vi "Phase_calculator_one_mask.vi"(9 "User-defined phase":dbl=4.0 format="%#_13g", 10 "User-defined Amplitude":dbl=0.3, 11 "Pixel":dbl=400.0) -> (0 "Voltage B Output":dbl=3921.0, 3 "Voltage A Output":dbl=1204.0)   [LabVIEW 2016]
uses:
  <vilib>/Utility/file.llb/Read Delimited Spreadsheet (DBL).vi
panel:
  out "Phase B Output 2":dbl=2.961 format="%#_8g"
  out "Voltage B Output 2":dbl=3921.0
  out "Amplitude Output 2":dbl=0.27793470017986477
  out "Phase Output 2":dbl=3.9764999999999997
  out "Voltage A Output 2":dbl=1204.0
  out "Phase A Output 2":dbl=4.992 format="%#_8g"
  in  "User-defined  Phi B":dbl=0.3
  out "arccos(A) 2":dbl=0.9911565864311924
  in  "User-defined Amplitude 2":dbl=0.3
  in  "Mask B phase output":cluster{"all rows":dbl[], "all rows":dbl[]}
  in  "Mask A phase output":cluster{"all rows":dbl[], "all rows":dbl[]}
  out "Amplitude Output":dbl=0.27793470017986477
  out "Phase Output":dbl=3.9764999999999997
  out "Phase A Output":dbl=4.992 format="%#_8g"
  out "Phase B Output":dbl=2.961 format="%#_8g"
  out "arccos(A)":dbl=0.9911565864311924
  in  "Mask B data string":string="G:\\My Drive\\ansom\\Data\\THz 1\\pulse shaping\\SLM calibration 5 August 2021\\Mask_B_phase_voltage\\Mask_B_phase_pixel_"
  in  "Mask A data string":string="G:\\My Drive\\ansom\\Data\\THz 1\\pulse shaping\\SLM calibration 5 August 2021\\Mask_A_phase_voltage\\Mask_A_phase_pixel_"
  out "Mask B Phase":cluster{"Ramp Pattern":dbl[], "phase out":dbl[]}(graph)
  out "Mask A Phase":cluster{"Ramp Pattern":dbl[], "phase out":dbl[]}(graph)
  in  "OK":bool
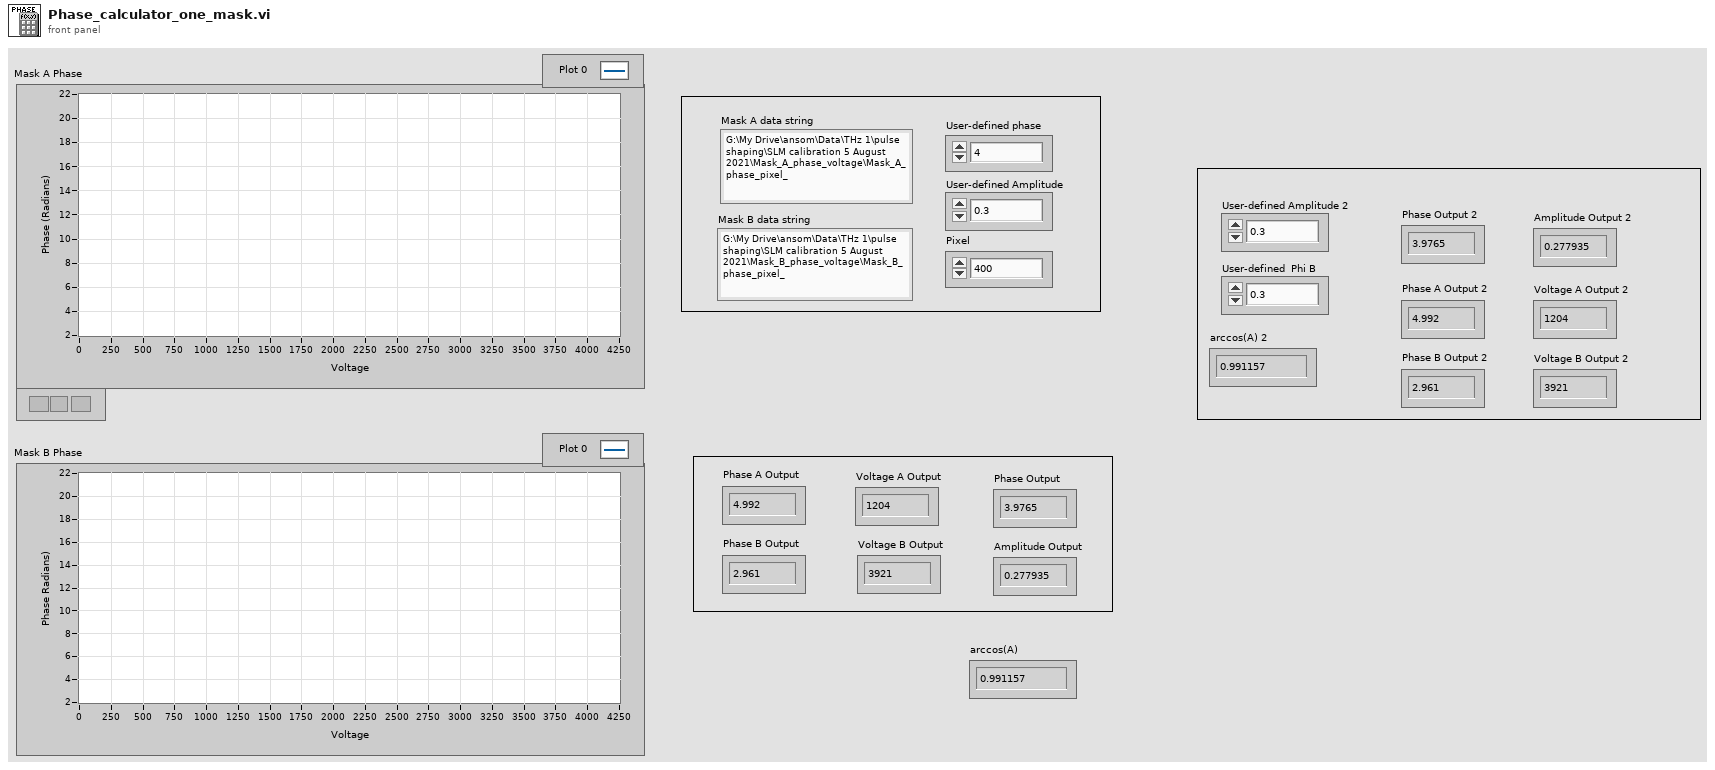
[diagram p1: front panel]
types:
  T1 = enum32{"Invalid", "Standard", "Closed", "Hidden", "Minimized", "Maximized"}
  T2 = enum32{"invalid app kind", "Development System", "Run Time System", "Student Edition", "Embedded LabVIEW", "Evaluation", "Custom"}
  T3 = cluster{"Core":cluster{"Current VI Reference":refnum<vi>, "Close Panel on Exit?":bool}, "Mask A phase output":cluster{"all rows":dbl[], "all rows":dbl[]}, "Mask B phase output":cluster{"all rows":dbl[], "all rows":dbl[]}}
  T4 = cluster{"Current VI Reference":refnum<vi>, "Close Panel on Exit?":bool}
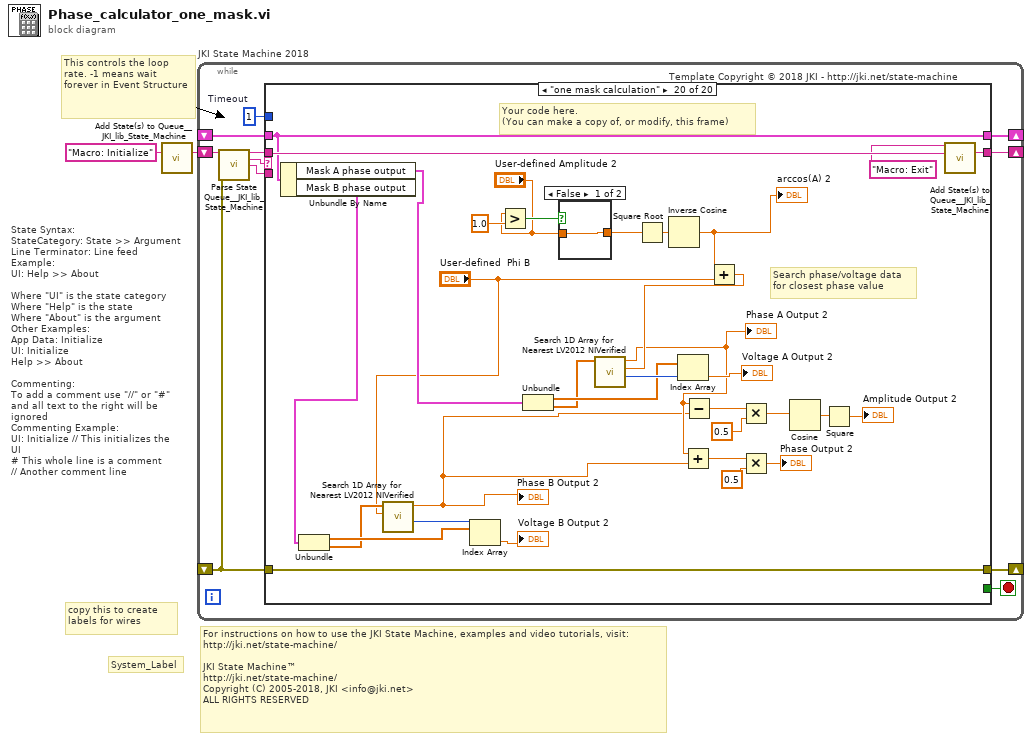
[diagram p0: block diagram]
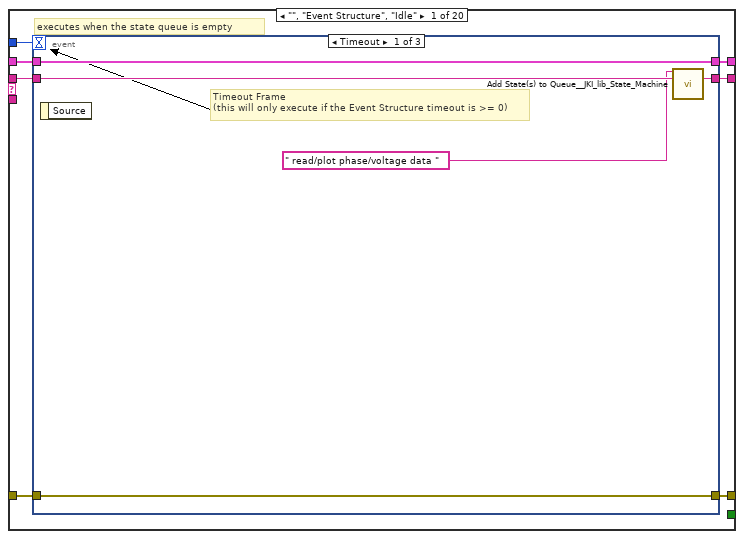
[diagram p2: hidden frame]
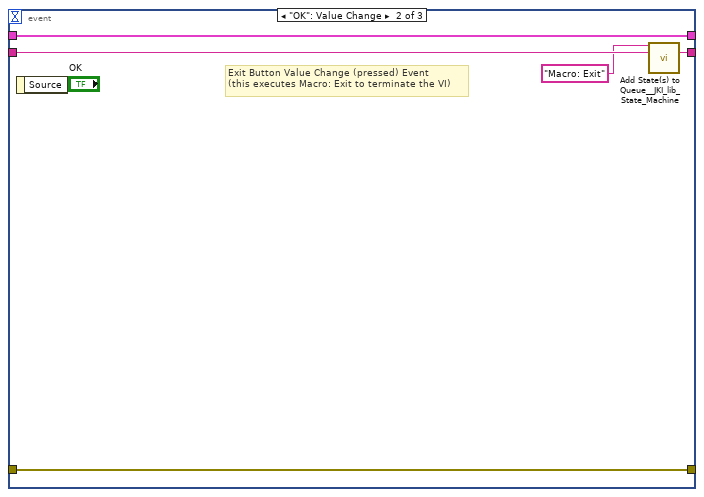
[diagram p3: hidden frame]
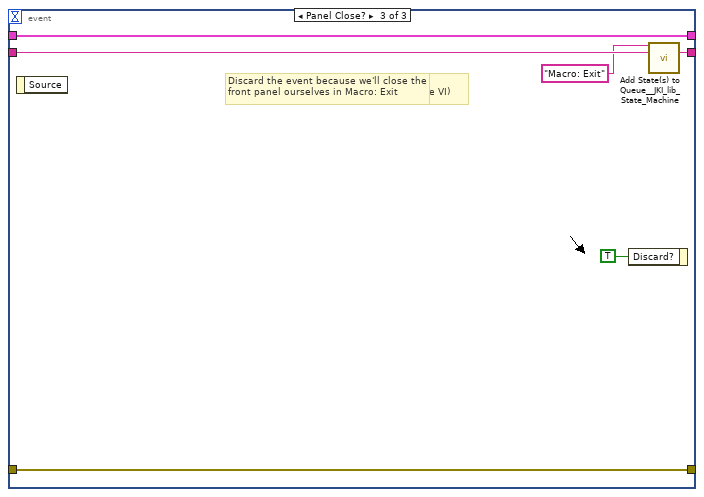
[diagram p4: hidden frame]
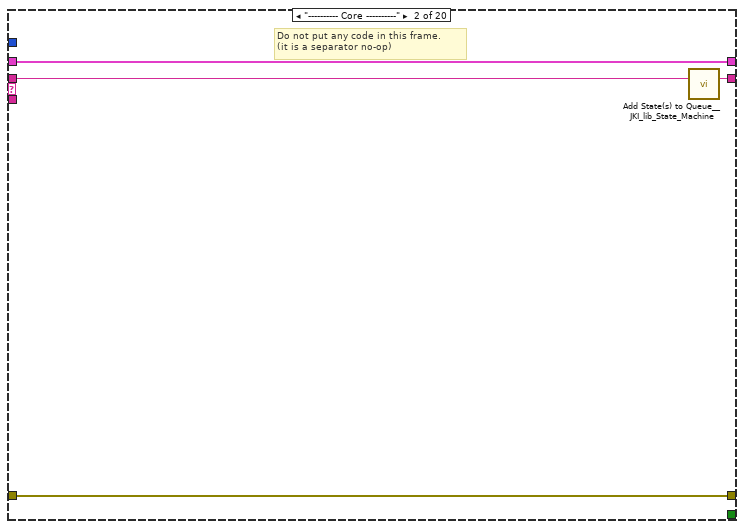
[diagram p5: hidden frame]
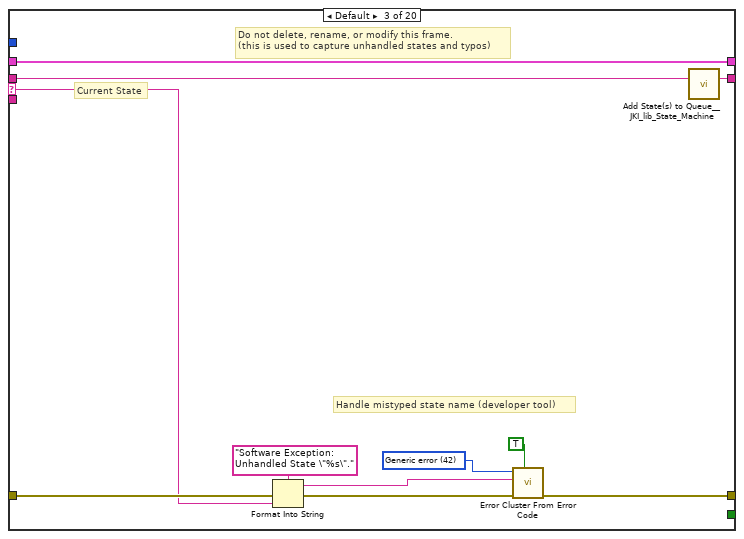
[diagram p6: hidden frame]
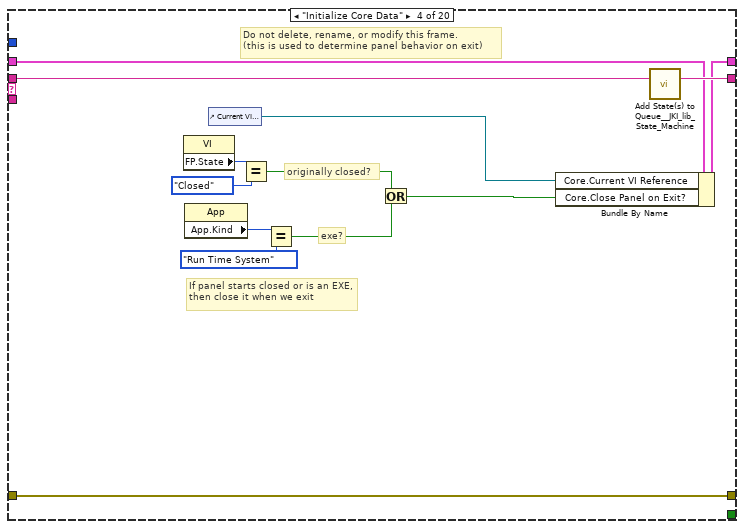
[diagram p7: hidden frame]
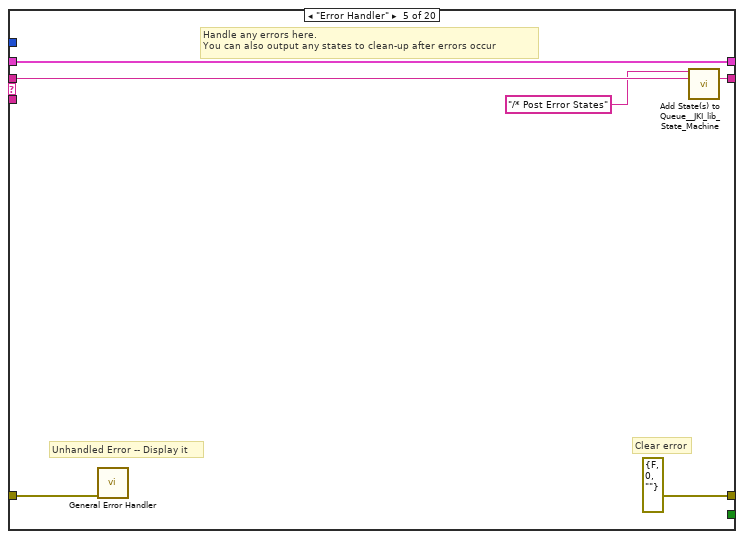
[diagram p8: hidden frame]
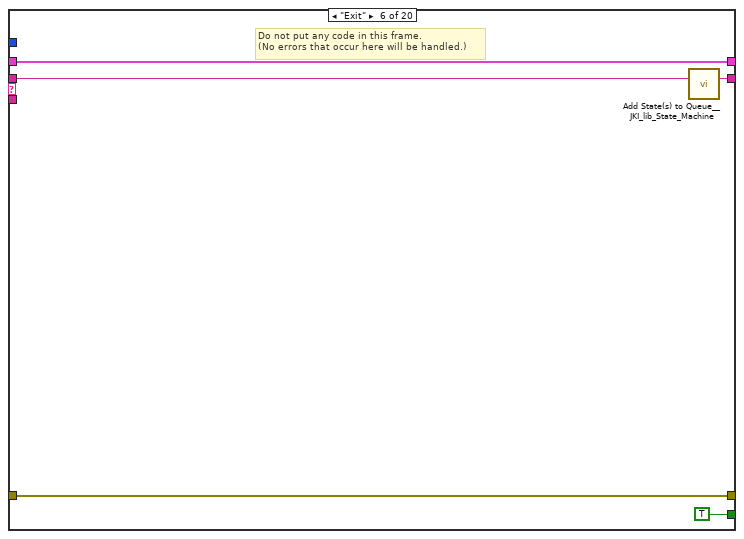
[diagram p9: hidden frame]
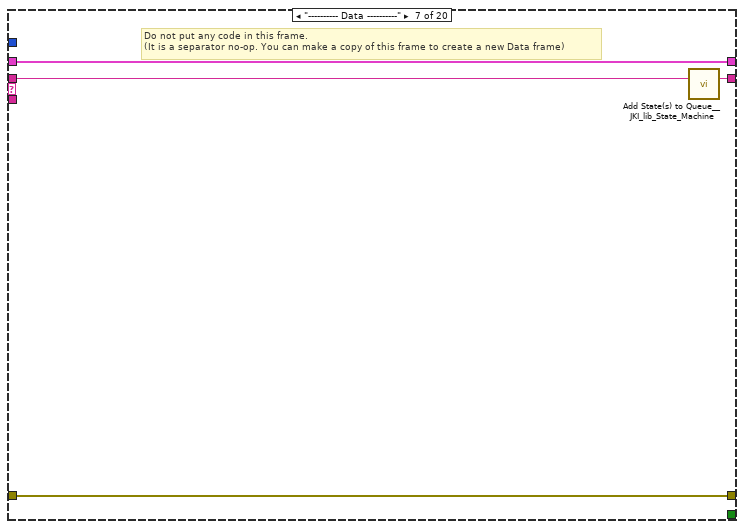
[diagram p10: hidden frame]
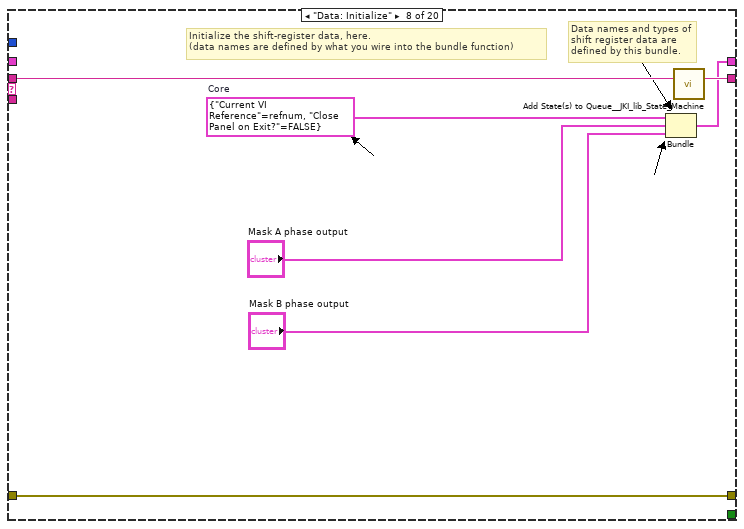
[diagram p11: hidden frame]
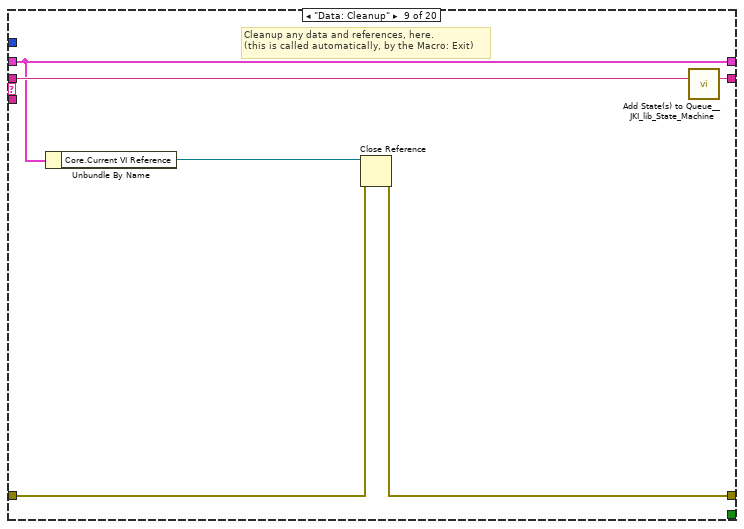
[diagram p12: hidden frame]
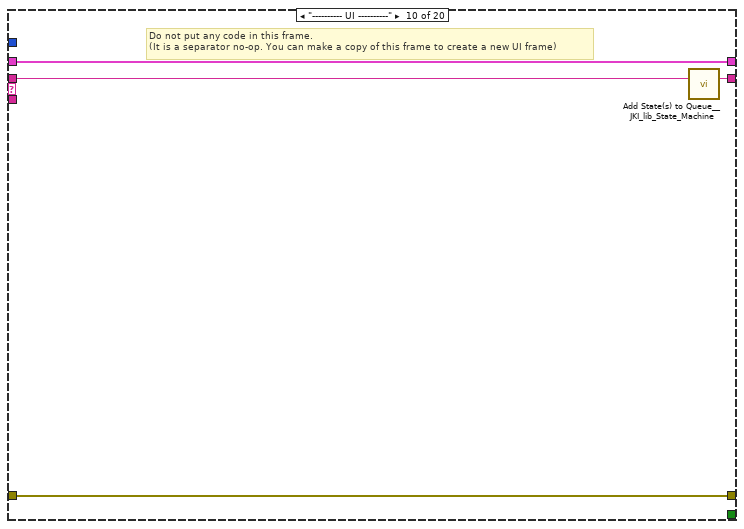
[diagram p13: hidden frame]
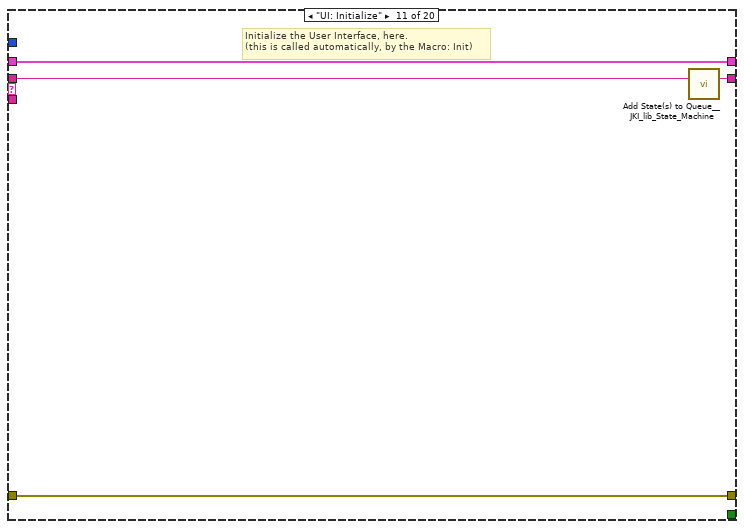
[diagram p14: hidden frame]
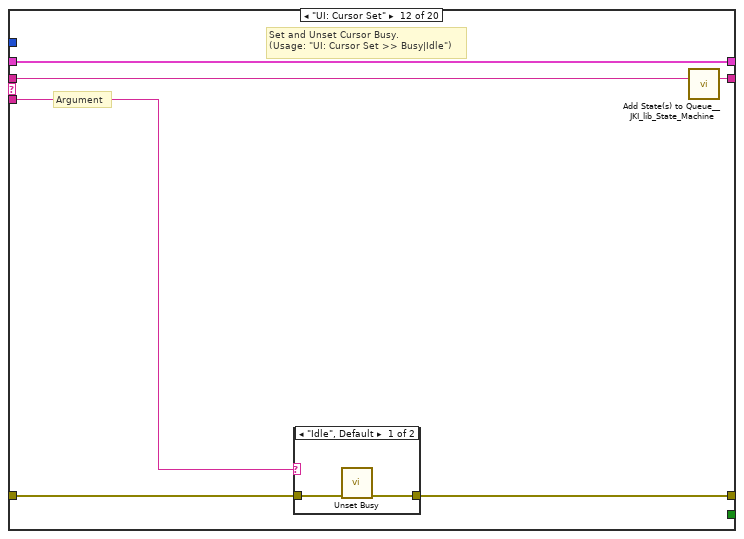
[diagram p15: hidden frame]
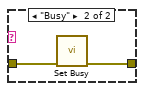
[diagram p16: hidden frame]
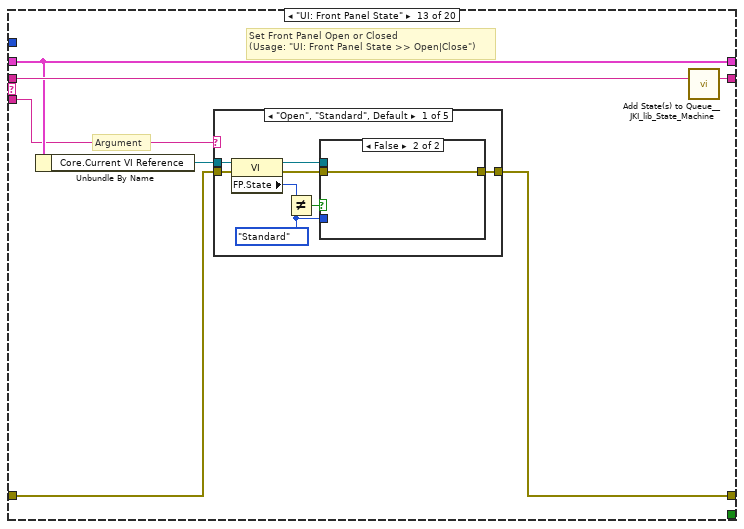
[diagram p17: hidden frame]
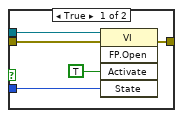
[diagram p18: hidden frame]
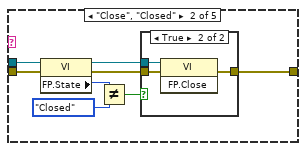
[diagram p19: hidden frame]
diagram:
  # "For instructions on how to use the JKI State Machine, examples and video tutorials, visit:\nhttp://jki.net/state-machine/\n\nJKI State Machine™\nhttp://jki.net/state-machine/\nCopyright (C) 2005-2018, JKI <info@jki.net>\nALL RIGHTS RESERVED"
  # "State Syntax:\nStateCategory: State >> Argument\nLine Terminator: Line feed\nExample:\nUI: Help >> About\n\nWhere \"UI\" is the state category\nWhere \"Help\" is the state\nWhere \"About\" is the argument\nOther Examples:\nApp Data: Initialize\nUI: Initialize\nHelp >> About\n\nCommenting:\nTo add a comment use \"//\" or \"#\" and all text to the right will be ignored\nCommenting Example:\nUI: Initialize // This initializes the UI\n# This whole line is a comment\n// Another comment line"
  # "copy this to create labels for wires"
  # "This controls the loop rate. -1 means wait forever in Event Structure"
  # "System_Label"
  n1 = call <vilib>:"Add State(s) to Queue__JKI_lib_State_Machine.vi"("State(s) in (\"\")"="Macro: Initialize") -> ("States Out"=w2:string)  [unwired: 14 in]
  n2 = while "JKI State Machine 2018" {
    shift-right: [w6] -> _
    shift-left: _ -> [w5]
    shift-right: [w9] -> _
    shift-left: _ -> [w3]
    shift-right: [w8] -> _
    shift-left: w2 -> [w10]
    stop <- w7 stop-if-true
    w4 = 1  # Timeout
    # "Template Copyright © 2018 JKI - http://jki.net/state-machine"
    n3 = call <vilib>:"Parse State Queue__JKI_lib_State_Machine.vi"("State Queue"=w10, "Error In (no error)"=w3) -> ("Remaining States"=w12:string, "Current State"=w13:string, "Arguments"=w11:string)  [unwired: 11 in]
    n4 = case shown="\"one mask calculation\"" w13 {
      selector: w13 -> [_ _ w41 _ _ _ _ _ _ _ _ _ _ _ _ _ _ _ _ _]
      tunnel: w12 -> [w20 w40 w45 w64 w70 w75 w79 w86 w92 w96 w100 w106 w117 w186 w191 w201 w205 w232 w271 w306]
      tunnel: w11 -> [_ _ _ _ _ _ _ _ _ _ _ w101 w111 _ _ _ _ _ _ _]
      tunnel: w5 -> [w18 w37 w43 w57 w67 w73 w76 _ w87 w93 w98 w104 w113 w183 w188 w198 w202 w211 w245 w303]
      tunnel: [w17 w38 w47 w61 errorcluster {"status"=FALSE, "code"=0, "source"=""} ("error out") w72 w77 w83 w88 w94 w97 w102 w114 w184 w189 w199 w203 w230 w269 w304] -> w9
      tunnel: w3 -> [w16 w38 w46 w61 w66 w72 w77 w83 w89 w94 w97 w103 w115 w184 w189 w199 w203 w230 w269 w304]
      tunnel: [w19 w39 w44 w63 w69 w74 w78 w85 w91 w95 w99 w105 w116 w185 w190 w200 w204 w231 w270 w305] -> w8
      tunnel: [_ _ _ _ _ TRUE _ _ _ _ _ _ _ _ _ _ _ _ _ _] -> w7
      tunnel: [w15 w37 w43 w62 w67 w73 w76 w84 w87 w93 w98 w104 w113 w183 w188 w198 w202 w210 w245 w303] -> w6
      tunnel: w4 -> [w14 _ _ _ _ _ _ _ _ _ _ _ _ _ _ _ _ _ _ _]
      frame "", "Event Structure", "Idle" {
        # "executes when the state queue is empty"
        n5 = event shown="[0] Timeout" {
          selector: _ -> [_ _ _]
          dyn-events: _ -> [_ _ _]
          timeout: w14 -> [_ _ _]
          tunnel: w20 -> [w25 w30 w36]
          tunnel: [w24 w29 w35] -> w19
          tunnel: w18 -> [w22 w27 w33]
          tunnel: [w23 w28 w34] -> w17
          tunnel: w16 -> [w23 w28 w34]
          tunnel: [w22 w27 w33] -> w15
          event Timeout {
            # "Timeout Frame\n(this will only execute if the Event Structure timeout is >= 0)"
            n6 = event-data() -> ()  [unwired: 1 in, 1 out]
            n7 = call <vilib>:"Add State(s) to Queue__JKI_lib_State_Machine.vi"("State(s) in Front (\"\")"=" read/plot phase/voltage data ", "State(s) in (\"\")"=w25) -> ("States Out"=w24:string)  [unwired: 13 in]
          }
          event "OK": Value Change {
            # "Exit Button Value Change (pressed) Event\n(this executes Macro: Exit to terminate the VI)"
            n8 = event-data() -> ()  [unwired: 1 in, 1 out]
            n9 = call <vilib>:"Add State(s) to Queue__JKI_lib_State_Machine.vi"("State(s) in Front (\"\")"="Macro: Exit", "State(s) in (\"\")"=w30) -> ("States Out"=w29:string)  [unwired: 13 in]
          }
          event Panel Close? {
            # "Discard the event because we'll close the front panel ourselves in Macro: Exit"
            # "Close Panel button (pressed) Event\n(this executes Macro: Exit to terminate the VI)"
            n10 = event-data() -> ()  [unwired: 1 in, 1 out]
            n11 = event-data("Discard?"=TRUE) -> ()  [unwired: 1 in, 1 out]
            n12 = call <vilib>:"Add State(s) to Queue__JKI_lib_State_Machine.vi"("State(s) in Front (\"\")"="Macro: Exit", "State(s) in (\"\")"=w36) -> ("States Out"=w35:string)  [unwired: 13 in]
          }
        }
      }
      frame "---------- Core ----------" {
        # "Do not put any code in this frame.\n(it is a separator no-op)"
        n13 = call <vilib>:"Add State(s) to Queue__JKI_lib_State_Machine.vi"("State(s) in (\"\")"=w40) -> ("States Out"=w39:string)  [unwired: 14 in]
      }
      frame Default {
        w50 = 42 items=["No error", "Argument error", "Memory is full", "Out of zone", "End of file", "File already open", "Generic file I/O error", "File not found", "File permission error", "Disk is full", "Duplicate path", "Too many files open", "System feature not enabled", "Resource file not found", "Cannot add resource", "Resource not found", "Image not found", "Image memory error", "Pen does not exist", "Config type invalid", "Config token not found", "Config parse error", "Config memory error", "Bad external code format", "Bad external code offset", "External code not present", "Null window", "Destroy window error", "Null menu", "Print aborted", "Bad print record", "Print driver error", "Windows error during printing", "Memory error during printing", "Print dialog error", "Generic print error", "Invalid device refnum", "Device not found", "Device parameter error", "Device unit error", "Cannot open device", "Device call aborted", "Generic error", "Cancelled by user", "Object ID too low", "Object ID too high", "Object not in heap", "Unknown heap", "Unknown object (invalid DefProc)", "Unknown object (DefProc not in table)", "Message out of range", "Invalid (null) method", "Unknown message", "Manager call not supported", "Bad address", "Network operation in progress", "Network operation timed out", "Connection is busy", "Network attribute not supported", "Network error", "Address in use", "System out of memory", "Connection aborted", "Connection refused", "Not connected", "Already connected", "Connection closed", "Initialization error (interapplication manager)", "Bad occurrence", "Wait on unbound occurrence handler", "Occurrence queue overflow", "Datalog type conflict", "Unused", "Unrecognized type (interapplication manager)", "Memory corrupt", "Failed to make temporary DLL", "Old CIN version", "Drag socket not found", "Failed to load drop-object", "Failed to register OLE object", "Failed to release OLE object", "Format specifier type mismatch", "Unknown format specifier", "Too few format specifiers", "Too many format specifiers", "Scan failed", "Newer CIN version", "Error converting to variant", "Runtime menu error", "Password tampered", "Variant attribute not found", "Incompatible variant data type", "Event data is not available", "Event Store is not present", "Occurrence is not found", "Event Queue is not created", "Event info is not available", "Refnum passed is NULL", "Error retrieving Class GUID", "Error retrieving CoClass GUID", "Error retrieving TypeLib GUID.", "Bad built application magic bytes.", "Specific driver is different from the specific driver associated with the Logical Name.", "There is no session opened to the class driver.", "Max Error", "MAX - Error with config objects", "MAX - Error loading configuration", "MAX - Group not supported"]
        # "Current State"
        # "Do not delete, rename, or modify this frame.\n(this is used to capture unhandled states and typos)"
        # "Handle mistyped state name (developer tool)"
        n14 = Format Into String(format string="Software Exception: Unhandled State \"%s\"." ("message"), error in=w46, w41) -> (resulting string=w49:string, error out=w48:errorcluster)  [unwired: 1 in]
        n15 = call <vilib>:"Error Cluster From Error Code.vi"("show call chain? (False)"=TRUE, "error in (no error)"=w48, "error message (\"\")"=w49, "error code (0)"=w50) -> ("error out"=w47:errorcluster)  [unwired: 5 in]
        n16 = call <vilib>:"Add State(s) to Queue__JKI_lib_State_Machine.vi"("State(s) in (\"\")"=w45) -> ("States Out"=w44:string)  [unwired: 14 in]
      }
      frame "Initialize Core Data" {
        # "Do not delete, rename, or modify this frame.\n(this is used to determine panel behavior on exit)"
        # "originally closed?"
        # "exe?"
        # "If panel starts closed or is an EXE, then close it when we exit"
        n17 = property class="VI"() -> ("FP.State"=w54:T1)  [unwired: 2 in, 2 out]
        n18 = property class="App"() -> ("App.Kind"=w60:T2)  [unwired: 2 in, 2 out]
        n19 = control-ref of="Current VI Reference"() -> (w55:refnum<vi>)
        n20 = Equal?(x=w54, y=T1."Closed" ("Front Panel Window:State")) -> (x = y?=w52:bool)
        n21 = Equal?(x=w60, y=T2."Run Time System" ("Application:Kind")) -> (x = y?=w58:bool)
        n22 = Or(x=w52, y=w58) -> (x .or. y?=w56:bool)
        n23 = Bundle By Name(cluster=w57, "Core.Current VI Reference"=w55, "Core.Close Panel on Exit?"=w56) -> (w62:T3)
        n24 = call <vilib>:"Add State(s) to Queue__JKI_lib_State_Machine.vi"("State(s) in (\"\")"=w64) -> ("States Out"=w63:string)  [unwired: 14 in]
      }
      frame "Error Handler" {
        # "Unhandled Error -- Display it"
        # "Handle any errors here.\nYou can also output any states to clean-up after errors occur"
        # "Clear error"
        n25 = call <vilib>:"General Error Handler.vi"("error in (no error)"=w66) -> ()  [unwired: 10 in, 5 out]
        n26 = call <vilib>:"Add State(s) to Queue__JKI_lib_State_Machine.vi"("State(s) in Front (\"\")"="/* Post Error States", "State(s) in (\"\")"=w70) -> ("States Out"=w69:string)  [unwired: 13 in]
      }
      frame "Exit" {
        # "Do not put any code in this frame.\n(No errors that occur here will be handled.)"
        n27 = call <vilib>:"Add State(s) to Queue__JKI_lib_State_Machine.vi"("State(s) in (\"\")"=w75) -> ("States Out"=w74:string)  [unwired: 14 in]
      }
      frame "---------- Data ----------" {
        # "Do not put any code in this frame.\n(It is a separator no-op. You can make a copy of this frame to create a new Data frame)"
        n28 = call <vilib>:"Add State(s) to Queue__JKI_lib_State_Machine.vi"("State(s) in (\"\")"=w79) -> ("States Out"=w78:string)  [unwired: 14 in]
      }
      frame "Data: Initialize" {
        w82 = T4 {"Current VI Reference"=refnum, "Close Panel on Exit?"=FALSE}  # Core
        # "Data names and types of shift register data are defined by this bundle."
        # "Initialize the shift-register data, here.\n(data names are defined by what you wire into the bundle function)"
        n29 = Bundle("Core"=w82, "Mask A phase output"="Mask A phase output", "Mask B phase output"="Mask B phase output") -> (w84:T3)  [unwired: 1 in]
        n30 = call <vilib>:"Add State(s) to Queue__JKI_lib_State_Machine.vi"("State(s) in (\"\")"=w86) -> ("States Out"=w85:string)  [unwired: 14 in]
      }
      frame "Data: Cleanup" {
        # "Cleanup any data and references, here.\n(this is called automatically, by the Macro: Exit)"
        n31 = Unbundle By Name(w87) -> ("Core.Current VI Reference"=w90:refnum<vi>)
        n32 = Close Reference(reference=w90, error in (no error)=w89) -> (error out=w88:errorcluster)
        n33 = call <vilib>:"Add State(s) to Queue__JKI_lib_State_Machine.vi"("State(s) in (\"\")"=w92) -> ("States Out"=w91:string)  [unwired: 14 in]
      }
      frame "---------- UI ----------" {
        # "Do not put any code in this frame.\n(It is a separator no-op. You can make a copy of this frame to create a new UI frame)"
        n34 = call <vilib>:"Add State(s) to Queue__JKI_lib_State_Machine.vi"("State(s) in (\"\")"=w96) -> ("States Out"=w95:string)  [unwired: 14 in]
      }
      frame "UI: Initialize" {
        # "Initialize the User Interface, here.\n(this is called automatically, by the Macro: Init)"
        n35 = call <vilib>:"Add State(s) to Queue__JKI_lib_State_Machine.vi"("State(s) in (\"\")"=w100) -> ("States Out"=w99:string)  [unwired: 14 in]
      }
      frame "UI: Cursor Set" {
        # "Argument"
        # "Set and Unset Cursor Busy.\n(Usage: \"UI: Cursor Set >> Busy|Idle\")"
        n36 = case shown="\"Idle\", Default" w101 {
          tunnel: w103 -> [w108 w110]
          tunnel: [w107 w109] -> w102
          frame "Idle", Default {
            n37 = call <vilib>:"Unset Busy.vi"("error in (no error)"=w108) -> ("error out"=w107:errorcluster)  [unwired: 10 in]
          }
          frame "Busy" {
            n38 = call <vilib>:"Set Busy.vi"("error in (no error)"=w110) -> ("error out"=w109:errorcluster)  [unwired: 9 in, 1 out]
          }
        }
        n39 = call <vilib>:"Add State(s) to Queue__JKI_lib_State_Machine.vi"("State(s) in (\"\")"=w106) -> ("States Out"=w105:string)  [unwired: 14 in]
      }
      frame "UI: Front Panel State" {
        # "Argument"
        # "Set Front Panel Open or Closed\n(Usage: \"UI: Front Panel State >> Open|Close\")"
        n40 = Unbundle By Name(w113) -> ("Core.Current VI Reference"=w112:refnum<vi>)
        n41 = case shown="\"Open\", \"Standard\", Default" w111 {
          tunnel: w115 -> [w123 w138 w149 w162 w175]
          tunnel: [w125 w139 w151 w164 w177] -> w114
          tunnel: w112 -> [w124 w136 w150 w163 w176]
          frame "Open", "Standard", Default {
            w118 = T1."Standard" ("State")
            n42 = property class="VI"(reference=w124, error in=w123) -> (reference out=w121:refnum<vi>, error out=w122:errorcluster, "FP.State"=w120:T1)
            n43 = Not Equal?(x=w120, y=w118) -> (x != y?=w119:bool)
            n44 = case shown="False" w119 {
              tunnel: [w129 w131] -> w125
              tunnel: w122 -> [w128 w131]
              tunnel: w121 -> [w127 _]
              tunnel: w118 -> [w126 _]
              frame True {
                n45 = invoke class="VI" method="FP.Open"(reference=w127, error in=w128, "Activate"=TRUE, "State"=w126) -> (error out=w129:errorcluster)  [unwired: 1 in, 4 out]
              }
              frame False {
              }
            }
          }
          frame "Close", "Closed" {
            n46 = property class="VI"(reference=w136, error in=w138) -> (reference out=w135:refnum<vi>, error out=w137:errorcluster, "FP.State"=w133:T1)
            n47 = Not Equal?(x=w133, y=T1."Closed" ("Front Panel Window:State")) -> (x != y?=w132:bool)
            n48 = case shown="True" w132 {
              tunnel: [w140 w143] -> w139
              tunnel: w137 -> [w140 w142]
              tunnel: w135 -> [_ w141]
              frame False {
              }
              frame True {
                n49 = invoke class="VI" method="FP.Close"(reference=w141, error in=w142) -> (error out=w143:errorcluster)  [unwired: 1 in, 2 out]
              }
            }
          }
          frame "Hidden", "Hide" {
            w144 = T1."Hidden" ("State")
            n50 = property class="VI"(reference=w150, error in=w149) -> (reference out=w147:refnum<vi>, error out=w148:errorcluster, "FP.State"=w146:T1)
            n51 = Not Equal?(x=w146, y=w144) -> (x != y?=w145:bool)
            n52 = case shown="True" w145 {
              tunnel: [w155 w156] -> w151
              tunnel: w148 -> [w154 w156]
              tunnel: w147 -> [w153 _]
              tunnel: w144 -> [w152 _]
              frame True {
                n53 = invoke class="VI" method="FP.Open"(reference=w153, error in=w154, "State"=w152) -> (error out=w155:errorcluster)  [unwired: 2 in, 4 out]
              }
              frame False {
              }
            }
          }
          frame "Minimize", "Minimized" {
            w157 = T1."Minimized" ("State")
            n54 = property class="VI"(reference=w163, error in=w162) -> (reference out=w160:refnum<vi>, error out=w161:errorcluster, "FP.State"=w159:T1)
            n55 = Not Equal?(x=w159, y=w157) -> (x != y?=w158:bool)
            n56 = case shown="True" w158 {
              tunnel: [w168 w169] -> w164
              tunnel: w161 -> [w167 w169]
              tunnel: w160 -> [w166 _]
              tunnel: w157 -> [w165 _]
              frame True {
                n57 = invoke class="VI" method="FP.Open"(reference=w166, error in=w167, "State"=w165) -> (error out=w168:errorcluster)  [unwired: 2 in, 4 out]
              }
              frame False {
              }
            }
          }
          frame "Maximize", "Maximized" {
            w170 = T1."Maximized" ("State")
            n58 = property class="VI"(reference=w176, error in=w175) -> (reference out=w173:refnum<vi>, error out=w174:errorcluster, "FP.State"=w172:T1)
            n59 = Not Equal?(x=w172, y=w170) -> (x != y?=w171:bool)
            n60 = case shown="True" w171 {
              tunnel: [w181 w182] -> w177
              tunnel: w174 -> [w180 w182]
              tunnel: w173 -> [w179 _]
              tunnel: w170 -> [w178 _]
              frame True {
                n61 = invoke class="VI" method="FP.Open"(reference=w179, error in=w180, "State"=w178) -> (error out=w181:errorcluster)  [unwired: 2 in, 4 out]
              }
              frame False {
              }
            }
          }
        }
        n62 = call <vilib>:"Add State(s) to Queue__JKI_lib_State_Machine.vi"("State(s) in (\"\")"=w117) -> ("States Out"=w116:string)  [unwired: 14 in]
      }
      frame "---------- Macro ----------" {
        # "Do not put any code in this frame.\n(It is a separator no-op. You can make a copy of this frame to create a new Macro frame)"
        n63 = call <vilib>:"Add State(s) to Queue__JKI_lib_State_Machine.vi"("State(s) in (\"\")"=w186) -> ("States Out"=w185:string)  [unwired: 14 in]
      }
      frame "Macro: Initialize" {
        w187 = "Data: Initialize\nInitialize Core Data\nUI: Initialize\nUI: Front Panel State >> Open"  # Data: Initialize Initialize Core Data UI: Initialize UI: Front Panel State >> Open
        # "Initialization Macro\n(This is called once, when the VI starts)"
        n64 = call <vilib>:"Add State(s) to Queue__JKI_lib_State_Machine.vi"("State(s) in Front (\"\")"=w187, "State(s) in (\"\")"=w191) -> ("States Out"=w190:string)  [unwired: 13 in]
      }
      frame "Macro: Exit" {
        # "Exit Macro\n(This is called once, when the VI exits)"
        n65 = Unbundle By Name(w198) -> ("Core.Close Panel on Exit?"=w197:bool)
        n66 = Select(t="UI: Front Panel State >> Close", s=w197, f="") -> (s? t:f=w194:string)
        n67 = call <vilib>:"Add State(s) to Queue__JKI_lib_State_Machine.vi"("State(s) in (\"\")"=w194, "State(s) at Back (\"\")"="Data: Cleanup\nExit") -> ("States Out"=w192:string)  [unwired: 13 in]
        n68 = call <vilib>:"Add State(s) to Queue__JKI_lib_State_Machine.vi"("State(s) in Front (\"\")"=w192, "State(s) in (\"\")"=w201) -> ("States Out"=w200:string)  [unwired: 13 in]
      }
      frame "---------- New Category ----------" {
        # "Template Separator\n(You can make a copy of, or modify, this frame)"
        n69 = call <vilib>:"Add State(s) to Queue__JKI_lib_State_Machine.vi"("State(s) in (\"\")"=w205) -> ("States Out"=w204:string)  [unwired: 14 in]
      }
      frame "read/plot phase/voltage data" {
        # "Plot phase/voltage data"
        # "Read voltage/phase curve data from file"
        # "Your code here.\n(You can make a copy of, or modify, this frame)"
        n70 = Number To Decimal String(number="Pixel") -> (decimal integer string=w220:string)  [unwired: 1 in]
        n71 = Number To Decimal String(number="Pixel") -> (decimal integer string=w221:string)  [unwired: 1 in]
        n72 = Concatenate Strings("Mask B data string", w220) -> (w219:string)
        n73 = String To Path(string=w219) -> (path=w218:path)
        n74 = call-poly <vilib>:"Read Delimited Spreadsheet.vi"("file path (dialog if empty)"=w218) -> ("all rows"=w227:dbl[][])  [unwired: 9 in, 5 out]
        n75 = Concatenate Strings("Mask A data string", w221) -> (w217:string)
        n76 = String To Path(string=w217) -> (path=w216:path)
        n77 = call-poly <vilib>:"Read Delimited Spreadsheet.vi"("file path (dialog if empty)"=w216) -> ("all rows"=w226:dbl[][])  [unwired: 9 in, 5 out]
        n78 = Index Array(array=w226, index (col)=0) -> (element=w222:dbl[])  [unwired: 1 in]
        n79 = Index Array(array=w227, index (col)=0) -> (element=w224:dbl[])  [unwired: 1 in]
        n80 = Index Array(array=w226, index (col)=1) -> (element=w223:dbl[])  [unwired: 1 in]
        n81 = Index Array(array=w227, index (col)=1) -> (element=w225:dbl[])  [unwired: 1 in]
        n82 = Bundle("all rows"=w222, "all rows"=w223) -> (w209:cluster{"all rows":dbl[], "all rows":dbl[]})  [unwired: 1 in]
        n83 = Bundle("all rows"=w224, "all rows"=w225) -> (w208:cluster{"all rows":dbl[], "all rows":dbl[]})  [unwired: 1 in]
        n84 = disable-structure shown="Disabled" {
          disable-tunnel: w209 -> [w234 _]
          disable-tunnel: w208 -> [w233 _]
          frame Disabled {
            "Mask A Phase" <- w234
            "Mask B Phase" <- w233
          }
          frame Enabled {
          }
        }
        n85 = Bundle By Name(cluster=w211, "Mask A phase output"=w209, "Mask B phase output"=w208) -> (w210:T3)
        n86 = call <vilib>:"Add State(s) to Queue__JKI_lib_State_Machine.vi"("State(s) in Front (\"\")"="one mask calculation", "State(s) in (\"\")"=w232) -> ("States Out"=w231:string)  [unwired: 13 in]
      }
      frame "Search phase/voltage for closest phase value" {
        w264 = 1.0
        # "Mask A phase phi_A"
        # "Mask B phase phi_B"
        # "Calculate overall phase and amplitude of pixel"
        # "Search phase/voltage data \nfor closest phase value"
        # "Your code here.\n(You can make a copy of, or modify, this frame)"
        n87 = Unbundle By Name(w245) -> ("Mask A phase output"=w244:cluster{"all rows":dbl[], "all rows":dbl[]}, "Mask B phase output"=w243:cluster{"all rows":dbl[], "all rows":dbl[]})
        n88 = Unbundle(w243) -> ("all rows"=w248:dbl[], "all rows"=w247:dbl[])
        n89 = Unbundle(w244) -> ("all rows"=w250:dbl[], "all rows"=w249:dbl[])
        n90 = Greater?(x="User-defined Amplitude", y=1.0) -> (0:w237:bool)
        n91 = case shown="False" w237 {
          tunnel: [w272 1.0] -> w236
          tunnel: "User-defined Amplitude" -> [w272 _]
          frame False {
          }
          frame True {
          }
        }
        n92 = Square Root(x=w236) -> (sqrt(x)=w240:dbl)
        n93 = Inverse Cosine(1:w240) -> (0:w267:dbl)
        "arccos(A)" <- w267
        n94 = Add(x="User-defined phase", y=w267) -> (x+y=w268:dbl)
        n95 = Subtract(x="User-defined phase", y=w267) -> (x-y=w266:dbl)
        n96 = Divide(x=w268, y=w264) -> (x/y=w242:dbl)
        n97 = call "Search 1D Array for Nearest LV2012 NIVerified.vi"("desired element"=w242, "1D Array"=w249) -> ("closest index"=w257:i32, "closest element"=w256:dbl)  [unwired: 8 in]
        "Phase A Output" <- w256
        n98 = Index Array(array=w250, index=w257) -> (element=→"Voltage A Output":dbl)
        n99 = Divide(x=w266, y=w264) -> (x/y=w246:dbl)
        n100 = call "Search 1D Array for Nearest LV2012 NIVerified.vi"("desired element"=w246, "1D Array"=w247) -> ("closest index"=w253:i32, "closest element"=w251:dbl)  [unwired: 8 in]
        "Phase B Output" <- w251
        n101 = Index Array(array=w248, index=w253) -> (element=→"Voltage B Output":dbl)
        n102 = Add(x=w256, y=w251) -> (x+y=w263:dbl)
        n103 = Subtract(x=w256, y=w251) -> (x-y=w259:dbl)
        n104 = Multiply(x=w259, y=0.5) -> (x*y=w258:dbl)
        n105 = Multiply(x=w263, y=0.5) -> (x*y=→"Phase Output":dbl)
        n106 = Cosine(x=w258) -> (cos(x)=w255:dbl)
        n107 = Square(x=w255) -> (x^2=→"Amplitude Output":dbl)
        n108 = call <vilib>:"Add State(s) to Queue__JKI_lib_State_Machine.vi"("State(s) in Front (\"\")"="Macro: Exit", "State(s) in (\"\")"=w271) -> ("States Out"=w270:string)  [unwired: 13 in]
      }
      frame "one mask calculation" {
        # "Search phase/voltage data \nfor closest phase value"
        # "Your code here.\n(You can make a copy of, or modify, this frame)"
        n109 = Unbundle By Name(w303) -> ("Mask A phase output"=w294:cluster{"all rows":dbl[], "all rows":dbl[]}, "Mask B phase output"=w278:cluster{"all rows":dbl[], "all rows":dbl[]})
        n110 = Unbundle(w278) -> ("all rows"=w280:dbl[], "all rows"=w279:dbl[])
        n111 = call "Search 1D Array for Nearest LV2012 NIVerified.vi"("desired element"="User-defined  Phi B", "1D Array"=w279) -> ("closest index"=w282:i32, "closest element"=w276:dbl)  [unwired: 8 in]
        "Phase B Output 2" <- w276
        n112 = Index Array(array=w280, index=w282) -> (element=→"Voltage B Output 2":dbl)
        n113 = Greater?(x="User-defined Amplitude 2", y=1.0) -> (0:w300:bool)
        n114 = Unbundle(w294) -> ("all rows"=w295:dbl[], "all rows"=w293:dbl[])
        n115 = case shown="False" w300 {
          tunnel: [w307 1.0] -> w275
          tunnel: "User-defined Amplitude 2" -> [w307 _]
          frame False {
          }
          frame True {
          }
        }
        n116 = Square Root(x=w275) -> (sqrt(x)=w274:dbl)
        n117 = Inverse Cosine(1:w274) -> (0:w298:dbl)
        "arccos(A) 2" <- w298
        n118 = Add(x=w298, y="User-defined  Phi B") -> (x+y=w292:dbl)
        n119 = call "Search 1D Array for Nearest LV2012 NIVerified.vi"("desired element"=w292, "1D Array"=w293) -> ("closest index"=w297:i32, "closest element"=w283:dbl)  [unwired: 8 in]
        "Phase A Output 2" <- w283
        n120 = Index Array(array=w295, index=w297) -> (element=→"Voltage A Output 2":dbl)
        n121 = Add(x=w283, y=w276) -> (x+y=w291:dbl)
        n122 = Subtract(x=w283, y=w276) -> (x-y=w287:dbl)
        n123 = Multiply(x=w287, y=0.5) -> (x*y=w286:dbl)
        n124 = Multiply(x=w291, y=0.5) -> (x*y=→"Phase Output 2":dbl)
        n125 = Cosine(x=w286) -> (cos(x)=w285:dbl)
        n126 = Square(x=w285) -> (x^2=→"Amplitude Output 2":dbl)
        n127 = call <vilib>:"Add State(s) to Queue__JKI_lib_State_Machine.vi"("State(s) in Front (\"\")"="Macro: Exit", "State(s) in (\"\")"=w306) -> ("States Out"=w305:string)  [unwired: 13 in]
      }
    }
  }
